vi "LS330_Set_Ramp.vi"(5 "Ramp Toggle":bool, 7 "error in":errorcluster, 8 "Ramp Rate":dbl, 9 "Heater":string(combo)="1", 10 "VISA resource name":refnum<visa-resource-name>) -> (0 "error out":errorcluster, 3 "VISA resource name out":refnum<visa-resource-name>)   [LabVIEW 2021]
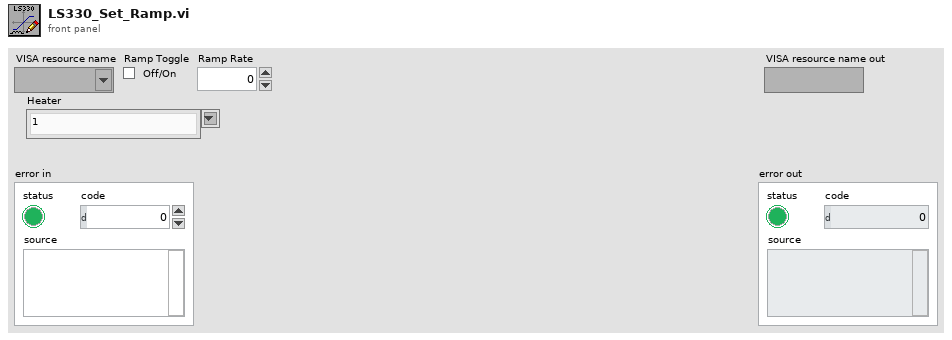
[diagram p1: front panel]
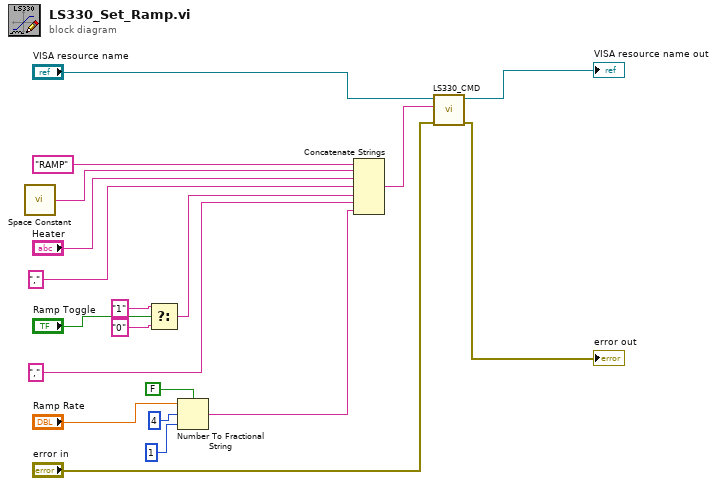
[diagram p0: block diagram]
diagram:
  n1 = call <vilib>:"Space Constant.vi"() -> ("String"=w17:string)
  n2 = Select(t="1", s="Ramp Toggle", f="0") -> (s? t:f=w7:string)
  n3 = Number To Fractional String(use system decimal point (T)=FALSE, number="Ramp Rate", width (-)=i16 4, precision (6)=i16 1) -> (F-format string=w2:string)
  n4 = Concatenate Strings("RAMP" ("string"), w17, "Heater", ",", w7, ",", w2) -> (w15:string)
  n5 = call "LS330_CMD.vi"("error in"="error in", "CMD"=w15, "VISA resource name"="VISA resource name") -> ("error out"=→"error out":errorcluster, "VISA resource name out"=→"VISA resource name out":refnum<visa-resource-name>)  [unwired: 7 in]
